vi "Superimpose Display A B Mode.vi"(8 "error in (no error)":errorcluster, 10 "SuperimposeDispDataA/B(T:On)":bool=TRUE, 11 "VISA resource name":refnum<visa-resource-name>) -> (0 "error out":errorcluster, 3 "VISA resource name out":refnum<visa-resource-name>)   [LabVIEW 2010, in "Agilent 4194.lvlib"]
doc: "This function is used for compare old and new data on instrument's display effective for A and B.\n\nNotes:\n\n(1) This function is valid for A - B setting only."
uses:
  <instrlib>/Agilent 4194/Agilent 4194.lvlib
panel:
  # "On\nOff"
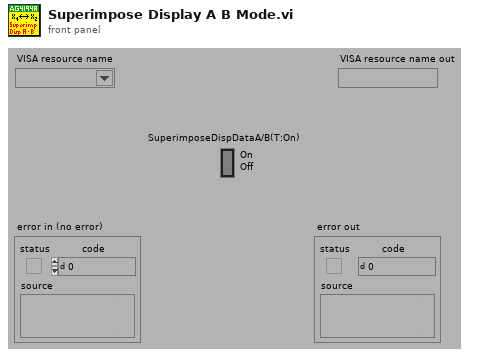
[diagram p1: front panel]
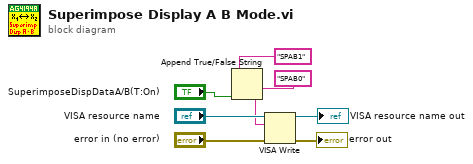
[diagram p0: block diagram]
diagram:
  n1 = Append True/False String(1:"SuperimposeDispDataA/B(T:On)", 2:"SPAB0", 3:"SPAB1") -> (0:w1:string)  [unwired: 1 in]
  n2 = VISA Write(VISA resource name="VISA resource name", write buffer=w1, error in (no error)="error in (no error)") -> (VISA resource name out=→"VISA resource name out":refnum<visa-resource-name>, error out=→"error out":errorcluster)  [unwired: 1 out]
